vi "buildsTimeStamp.vi"(1 "Select FORMAT":T1(ring)=enum."00M00D_00h00m", 4 "t0":timestamp, 6 "Include milli second?":bool) -> (15 "TimeStamp":string)   [LabVIEW 2022 SP3, in "stillnessHelper.lvclass"]
uses:
  stillnessHelper.lvclass
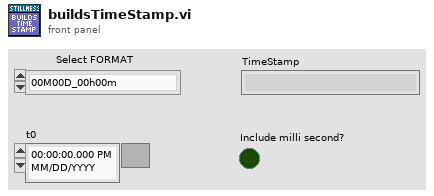
[diagram p1: front panel]
types:
  T1 = enum16{"Y00M00D00h00m00s00", "YYMMDD(hhmmss)", "00Y00M00D00h00m00s", "0000Y00M00D00h00m00s", "00M00D_00h00m", "0000-00-00 00h00m00s", "0000_00_00_00h00m00s", "00000000_000000", "000000_000000", "YYYY-MM-DD,hh:mm:ss"}
  T2 = typedef "LVDateTimeRec.ctl" = cluster{"fractional second":dbl, "second":i32, "minute":i32, "hour":i32, "day of month":i32, "month":i32, "year":i32, "day of week":i32, "day of year":i32, "DST":i32}
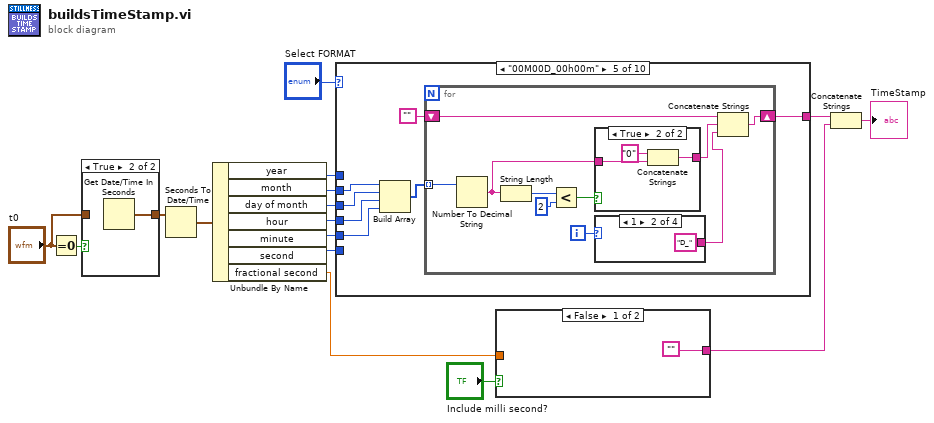
[diagram p0: block diagram]
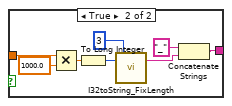
[diagram p2: hidden frame]
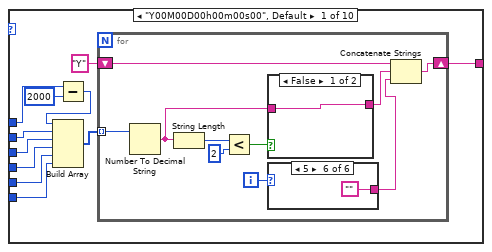
[diagram p4: hidden frame]
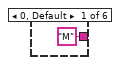
[diagram p5: hidden frame]
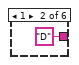
[diagram p6: hidden frame]
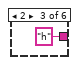
[diagram p7: hidden frame]
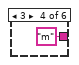
[diagram p8: hidden frame]
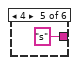
[diagram p9: hidden frame]
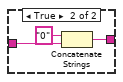
[diagram p10: hidden frame]
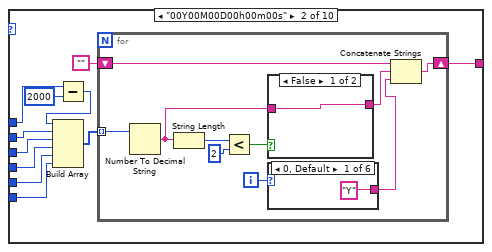
[diagram p11: hidden frame]
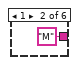
[diagram p12: hidden frame]
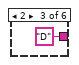
[diagram p13: hidden frame]
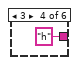
[diagram p14: hidden frame]
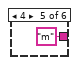
[diagram p15: hidden frame]
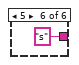
[diagram p16: hidden frame]
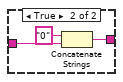
[diagram p17: hidden frame]
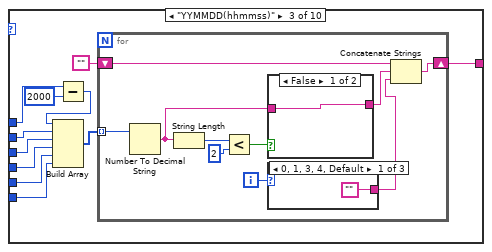
[diagram p18: hidden frame]
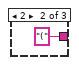
[diagram p19: hidden frame]
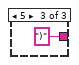
[diagram p20: hidden frame]
diagram:
  n1 = Equal To 0?(x="t0") -> (x = 0?=w9:bool)
  n2 = case shown="True" w9 {
    tunnel: [w17 w18] -> w7
    tunnel: "t0" -> [w17 _]
    frame False {
    }
    frame True {
      n3 = Get Date/Time In Seconds() -> (seconds since 1Jan1904=w18:timestamp)
    }
  }
  n4 = Seconds To Date/Time(time stamp (now)=w7) -> (date time rec=w6:T2)  [unwired: 1 in]
  n5 = Unbundle By Name(w6) -> ("year"=w15:i32, "month"=w14:i32, "day of month"=w13:i32, "hour"=w12:i32, "minute"=w11:i32, "second"=w10:i32, "fractional second"=w5:dbl)
  n6 = case shown="\"00M00D_00h00m\"" "Select FORMAT" {
    tunnel: w10 -> [w20 w52 w83 w112 _ w166 w195 w224 w253 w280]
    tunnel: w11 -> [w21 w53 w84 w113 w140 w167 w196 w225 w254 w281]
    tunnel: w12 -> [w22 w54 w85 w114 w141 w168 w197 w226 w255 w282]
    tunnel: w13 -> [w27 w58 w89 w115 w142 w169 w198 w227 w256 w283]
    tunnel: w14 -> [w28 w59 w90 w116 w143 w170 w199 w228 w257 w284]
    tunnel: w15 -> [w25 w57 w88 w109 _ w163 w192 w221 w250 w277]
    tunnel: [w19 w51 w82 w111 w139 w165 w194 w223 w252 w275] -> w3
    frame "Y00M00D00h00m00s00", Default {
      n7 = Subtract(x=w25, y=2000) -> (x-y=w23:i32)
      n8 = Build Array(w23, w28, w27, w22, w21, w20) -> (w29:i32[])
      n9 = for {
        tunnel: w29 -> [w35] mode=indexing
        shift-right: [w34] -> w19
        shift-left: "Y" -> [w33]
        i -> [w31]
        n10 = Number To Decimal String(number=w35) -> (decimal integer string=w39:string)  [unwired: 1 out]
        n11 = String Length(string=w39) -> (length=w36:i32)
        n12 = Less?(x=w36, y=2) -> (x < y?=w38:bool)
        n13 = case shown="False" w38 {
          tunnel: w39 -> [w46 w49]
          tunnel: [w46 w47] -> w32
          frame False {
          }
          frame True {
            n14 = Concatenate Strings("0" ("string"), w49) -> (w47:string)
          }
        }
        n15 = case shown="5" w31 {
          tunnel: ["M" "D" "h" "m" "s" ""] -> w30
          frame 0, Default {
          }
          frame 1 {
          }
          frame 2 {
          }
          frame 3 {
          }
          frame 4 {
          }
          frame 5 {
          }
        }
        n16 = Concatenate Strings(w33, w32, w30) -> (w34:string)
      }
    }
    frame "00Y00M00D00h00m00s" {
      n17 = Subtract(x=w57, y=2000) -> (x-y=w55:i32)
      n18 = Build Array(w55, w59, w58, w54, w53, w52) -> (w60:i32[])
      n19 = for {
        tunnel: w60 -> [w66] mode=indexing
        shift-right: [w65] -> w51
        shift-left: "" -> [w64]
        i -> [w62]
        n20 = Number To Decimal String(number=w66) -> (decimal integer string=w70:string)  [unwired: 1 out]
        n21 = String Length(string=w70) -> (length=w67:i32)
        n22 = Less?(x=w67, y=2) -> (x < y?=w69:bool)
        n23 = case shown="False" w69 {
          tunnel: w70 -> [w77 w80]
          tunnel: [w77 w78] -> w63
          frame False {
          }
          frame True {
            n24 = Concatenate Strings("0" ("string"), w80) -> (w78:string)
          }
        }
        n25 = case shown="0, Default" w62 {
          tunnel: ["Y" "M" "D" "h" "m" "s"] -> w61
          frame 0, Default {
          }
          frame 1 {
          }
          frame 2 {
          }
          frame 3 {
          }
          frame 4 {
          }
          frame 5 {
          }
        }
        n26 = Concatenate Strings(w64, w63, w61) -> (w65:string)
      }
    }
    frame "YYMMDD(hhmmss)" {
      n27 = Subtract(x=w88, y=2000) -> (x-y=w86:i32)
      n28 = Build Array(w86, w90, w89, w85, w84, w83) -> (w91:i32[])
      n29 = for {
        tunnel: w91 -> [w97] mode=indexing
        shift-right: [w96] -> w82
        shift-left: "" -> [w95]
        i -> [w93]
        n30 = Number To Decimal String(number=w97) -> (decimal integer string=w101:string)  [unwired: 1 out]
        n31 = String Length(string=w101) -> (length=w98:i32)
        n32 = Less?(x=w98, y=2) -> (x < y?=w100:bool)
        n33 = case shown="False" w100 {
          tunnel: w101 -> [w105 w108]
          tunnel: [w105 w106] -> w94
          frame False {
          }
          frame True {
            n34 = Concatenate Strings("0" ("string"), w108) -> (w106:string)
          }
        }
        n35 = case shown="0, 1, 3, 4, Default" w93 {
          tunnel: ["" "(" ")"] -> w92
          frame 0, 1, 3, 4, Default {
          }
          frame 2 {
          }
          frame 5 {
          }
        }
        n36 = Concatenate Strings(w95, w94, w92) -> (w96:string)
      }
    }
    frame "0000Y00M00D00h00m00s" {
      n37 = Build Array(w109, w116, w115, w114, w113, w112) -> (w117:i32[])
      n38 = for {
        tunnel: w117 -> [w123] mode=indexing
        shift-right: [w122] -> w111
        shift-left: "" -> [w121]
        i -> [w119]
        n39 = Number To Decimal String(number=w123) -> (decimal integer string=w127:string)  [unwired: 1 out]
        n40 = String Length(string=w127) -> (length=w124:i32)
        n41 = Less?(x=w124, y=2) -> (x < y?=w126:bool)
        n42 = case shown="False" w126 {
          tunnel: w127 -> [w134 w137]
          tunnel: [w134 w135] -> w120
          frame False {
          }
          frame True {
            n43 = Concatenate Strings("0" ("string"), w137) -> (w135:string)
          }
        }
        n44 = case shown="0, Default" w119 {
          tunnel: ["Y" "M" "D" "h" "m" "s"] -> w118
          frame 0, Default {
          }
          frame 1 {
          }
          frame 2 {
          }
          frame 3 {
          }
          frame 4 {
          }
          frame 5 {
          }
        }
        n45 = Concatenate Strings(w121, w120, w118) -> (w122:string)
      }
    }
    frame "00M00D_00h00m" {
      n46 = Build Array(w143, w142, w141, w140) -> (w144:i32[])
      n47 = for {
        tunnel: w144 -> [w150] mode=indexing
        shift-right: [w149] -> w139
        shift-left: "" -> [w148]
        i -> [w146]
        n48 = Number To Decimal String(number=w150) -> (decimal integer string=w154:string)  [unwired: 1 out]
        n49 = String Length(string=w154) -> (length=w151:i32)
        n50 = Less?(x=w151, y=2) -> (x < y?=w153:bool)
        n51 = case shown="True" w153 {
          tunnel: w154 -> [w159 w162]
          tunnel: [w159 w160] -> w147
          frame False {
          }
          frame True {
            n52 = Concatenate Strings("0" ("string"), w162) -> (w160:string)
          }
        }
        n53 = case shown="1" w146 {
          tunnel: ["M" "D_" "h" "m"] -> w145
          frame 0, Default {
          }
          frame 1 {
          }
          frame 2 {
          }
          frame 3 {
          }
        }
        n54 = Concatenate Strings(w148, w147, w145) -> (w149:string)
      }
    }
    frame "0000-00-00 00h00m00s" {
      n55 = Build Array(w163, w170, w169, w168, w167, w166) -> (w171:i32[])
      n56 = for {
        tunnel: w171 -> [w177] mode=indexing
        shift-right: [w176] -> w165
        shift-left: "" -> [w175]
        i -> [w173]
        n57 = Number To Decimal String(number=w177) -> (decimal integer string=w181:string)  [unwired: 1 out]
        n58 = String Length(string=w181) -> (length=w178:i32)
        n59 = Less?(x=w178, y=2) -> (x < y?=w180:bool)
        n60 = case shown="True" w180 {
          tunnel: w181 -> [w188 w191]
          tunnel: [w188 w189] -> w174
          frame False {
          }
          frame True {
            n61 = Concatenate Strings("0" ("string"), w191) -> (w189:string)
          }
        }
        n62 = case shown="0, Default" w173 {
          tunnel: ["-" "-" " " "h" "m" "s"] -> w172
          frame 0, Default {
          }
          frame 1 {
          }
          frame 2 {
          }
          frame 3 {
          }
          frame 4 {
          }
          frame 5 {
          }
        }
        n63 = Concatenate Strings(w175, w174, w172) -> (w176:string)
      }
    }
    frame "YYYY-MM-DD,hh:mm:ss" {
      n64 = Build Array(w192, w199, w198, w197, w196, w195) -> (w200:i32[])
      n65 = for {
        tunnel: w200 -> [w206] mode=indexing
        shift-right: [w205] -> w194
        shift-left: "" -> [w204]
        i -> [w202]
        n66 = Number To Decimal String(number=w206) -> (decimal integer string=w210:string)  [unwired: 1 out]
        n67 = String Length(string=w210) -> (length=w207:i32)
        n68 = Less?(x=w207, y=2) -> (x < y?=w209:bool)
        n69 = case shown="True" w209 {
          tunnel: w210 -> [w217 w220]
          tunnel: [w217 w218] -> w203
          frame False {
          }
          frame True {
            n70 = Concatenate Strings("0" ("string"), w220) -> (w218:string)
          }
        }
        n71 = case shown="5" w202 {
          tunnel: ["-" "-" "," ":" ":" ""] -> w201
          frame 0, Default {
          }
          frame 1 {
          }
          frame 2 {
          }
          frame 3 {
          }
          frame 4 {
          }
          frame 5 {
          }
        }
        n72 = Concatenate Strings(w204, w203, w201) -> (w205:string)
      }
    }
    frame "0000_00_00_00h00m00s" {
      n73 = Build Array(w221, w228, w227, w226, w225, w224) -> (w229:i32[])
      n74 = for {
        tunnel: w229 -> [w235] mode=indexing
        shift-right: [w234] -> w223
        shift-left: "" -> [w233]
        i -> [w231]
        n75 = Number To Decimal String(number=w235) -> (decimal integer string=w239:string)  [unwired: 1 out]
        n76 = String Length(string=w239) -> (length=w236:i32)
        n77 = Less?(x=w236, y=2) -> (x < y?=w238:bool)
        n78 = case shown="True" w238 {
          tunnel: w239 -> [w246 w249]
          tunnel: [w246 w247] -> w232
          frame False {
          }
          frame True {
            n79 = Concatenate Strings("0" ("string"), w249) -> (w247:string)
          }
        }
        n80 = case shown="3" w231 {
          tunnel: ["_" "_" "_" "h" "m" "s"] -> w230
          frame 0, Default {
          }
          frame 1 {
          }
          frame 2 {
          }
          frame 3 {
          }
          frame 4 {
          }
          frame 5 {
          }
        }
        n81 = Concatenate Strings(w233, w232, w230) -> (w234:string)
      }
    }
    frame "00000000_000000" {
      n82 = Build Array(w250, w257, w256, w255, w254, w253) -> (w258:i32[])
      n83 = for {
        tunnel: w258 -> [w264] mode=indexing
        shift-right: [w263] -> w252
        shift-left: "" -> [w262]
        i -> [w260]
        n84 = Number To Decimal String(number=w264) -> (decimal integer string=w268:string)  [unwired: 1 out]
        n85 = String Length(string=w268) -> (length=w265:i32)
        n86 = Less?(x=w265, y=2) -> (x < y?=w267:bool)
        n87 = case shown="True" w267 {
          tunnel: w268 -> [w271 w274]
          tunnel: [w271 w272] -> w261
          frame False {
          }
          frame True {
            n88 = Concatenate Strings("0" ("string"), w274) -> (w272:string)
          }
        }
        n89 = case shown="0, Default" w260 {
          tunnel: ["" "_"] -> w259
          frame 0, Default {
          }
          frame 2 {
          }
        }
        n90 = Concatenate Strings(w262, w261, w259) -> (w263:string)
      }
    }
    frame "000000_000000" {
      n91 = Subtract(x=w277, y=2000) -> (x-y=w276:i32)
      n92 = Build Array(w276, w284, w283, w282, w281, w280) -> (w285:i32[])
      n93 = for {
        tunnel: w285 -> [w291] mode=indexing
        shift-right: [w290] -> w275
        shift-left: "" -> [w289]
        i -> [w287]
        n94 = Number To Decimal String(number=w291) -> (decimal integer string=w295:string)  [unwired: 1 out]
        n95 = String Length(string=w295) -> (length=w292:i32)
        n96 = Less?(x=w292, y=2) -> (x < y?=w294:bool)
        n97 = case shown="True" w294 {
          tunnel: w295 -> [w298 w301]
          tunnel: [w298 w299] -> w288
          frame False {
          }
          frame True {
            n98 = Concatenate Strings("0" ("string"), w301) -> (w299:string)
          }
        }
        n99 = case shown="0, Default" w287 {
          tunnel: ["" "_"] -> w286
          frame 0, Default {
          }
          frame 2 {
          }
        }
        n100 = Concatenate Strings(w289, w288, w286) -> (w290:string)
      }
    }
  }
  n101 = case shown="False" "Include milli second?" {
    tunnel: w5 -> [_ w310]
    tunnel: ["" w308] -> w2
    frame False {
    }
    frame True {
      n102 = Multiply(x=w310, y=1000.0) -> (x*y=w306:dbl)
      n103 = To Long Integer(number=w306) -> (32bit integer=w305:i32)
      n104 = call "I32toString_FixLength.vi"("I32"=w305, "Length (Nb Char)"=u8 3) -> ("String OUT"=w303:string)  [unwired: 17 in]
      n105 = Concatenate Strings("_" ("string"), w303) -> (w308:string)
    }
  }
  n106 = Concatenate Strings(w3, w2) -> (→"TimeStamp":string)
